vi "Config Field.vi"(4 "Error Messages (Message)":i32(ring)=1 items=["Code", "Message"], 5 "Sample (off)":bool, 6 "Voltage (on)":bool=TRUE, 7 "Frequency (on)":bool=TRUE, 8 "error in":errorcluster, 9 "Loss (9)":i32=9 min=0 max=9, 10 "Capacitance (9)":i32=9 min=0 max=9, 11 "VISA resource name":refnum<visa-resource-name>) -> (0 "error out":errorcluster, 3 "VISA resource name out":refnum<visa-resource-name>)   [LabVIEW 2016, in "Andeen-Hagerling 2550.lvlib"]
doc: "This VI configures which fields are sent to serial or GPIB ports. Also controls the number of significant digits reported for capacitance and/or loss measurements to the front panel and remote devices. Note that default parameter values correspond to the bridge default values and not the values assigned in <b>Default Instrument Setup.vi</b>."
uses:
  Andeen-Hagerling 2550.lvlib
panel:
  # "Field Parameters"
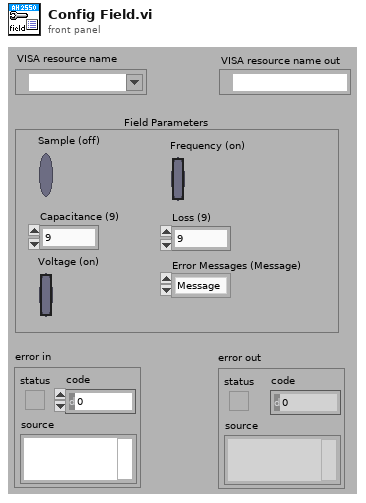
[diagram p1: front panel]
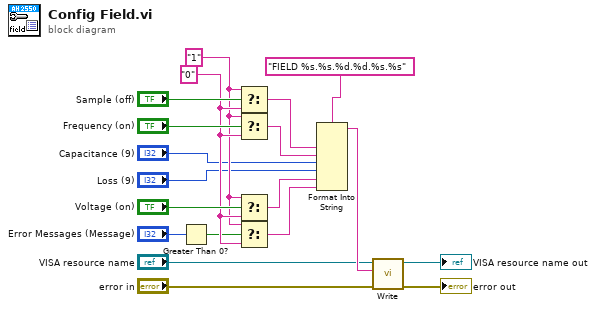
[diagram p0: block diagram]
diagram:
  w16 = "0"
  w15 = "1"
  n1 = Greater Than 0?(x="Error Messages (Message)") -> (x > 0?=w2:bool)
  n2 = Select(t=w15, s="Sample (off)", f=w16) -> (s? t:f=w14:string)
  n3 = Select(t=w15, s="Frequency (on)", f=w16) -> (s? t:f=w13:string)
  n4 = Select(t=w15, s="Voltage (on)", f=w16) -> (s? t:f=w10:string)
  n5 = Select(t=w15, s=w2, f=w16) -> (s? t:f=w9:string)
  n6 = Format Into String(format string="FIELD %s.%s.%d.%d.%s.%s", w14, w13, "Capacitance (9)", "Loss (9)", w10, w9) -> (resulting string=w7:string)  [unwired: 2 in, 1 out]
  n7 = call "Write.vi"("error in"="error in", "command"=w7, "VISA resource name"="VISA resource name") -> ("error out"=→"error out":errorcluster, "VISA resource name out"=→"VISA resource name out":refnum<visa-resource-name>)  [unwired: 7 in]
